vi "Test Drive OO.vi"() -> ()   [LabVIEW 2024]
uses:
  Ocean Optics Driver.lvclass
  Utilities/Fit/Peak Parameters.ctl
  Utilities/Fit/Multi-peak Parameters.ctl
  Ocean optics configuration.ctl
  LabActor/Recorders/Ruby Spectra/Ruby Spectra.lvclass
panel:
  in  "VISA resource name":refnum<visa-resource-name>="MayaPro"
  out "Spectral Waveform":T1(graph)
  in  "Ocean optics configuration":T2={"Integration time"=0.5, "Fit parameters"={"Function"=enum."Gauss", "Window width"=0.0, "Initial guess"={"Amplitude"=0.0, "Center"=690.0, "Width"=3.0}}, "Fit"=FALSE, "Auto-update params"=FALSE, "Save spectra"=FALSE, "Reference wavelengh"=694.123, "Background"=path ""} {"Reference wavelengh" format="%#_gnm"; "Fit parameters"."Initial guess"."Width" format="%#_gnm"; "Fit parameters"."Initial guess"."Center" format="%#_gnm"; "Fit parameters"."Window width" format="%#_6gnm"; "Integration time" format="%#_6ps"}
  in  "Device":string="MayaPro"
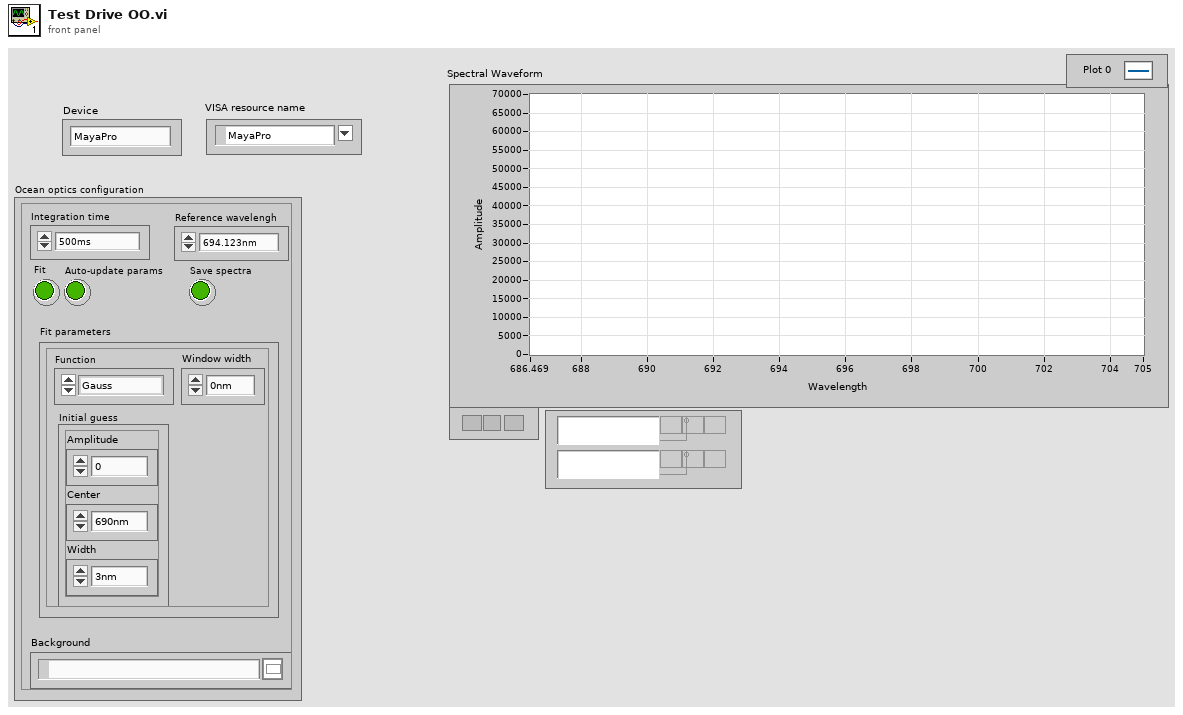
[diagram p1: front panel]
types:
  T1 = cluster{"Wavelength (nm)":dbl[], "Spectrum by Pixel Number":dbl[]}[]
  T2 = typedef "Ruby Spectra.lvclass/Ocean optics configuration.ctl" = cluster{"Integration time":dbl, "Fit parameters":T3, "Fit":bool, "Auto-update params":bool, "Save spectra":bool, "Reference wavelengh":dbl, "Background":path}
  T3 = typedef "Multi-peak Parameters.ctl" = cluster{"Function":enum16{"Gauss", "Lorentz"}, "Window width":dbl, "Initial guess":T4}
  T4 = typedef "Peak Parameters.ctl" = cluster{"Amplitude":dbl, "Center":dbl, "Width":dbl}
  T5 = cluster{"Wavelengths":dbl[], "Spectrum by Pixel Number":dbl[]}[]
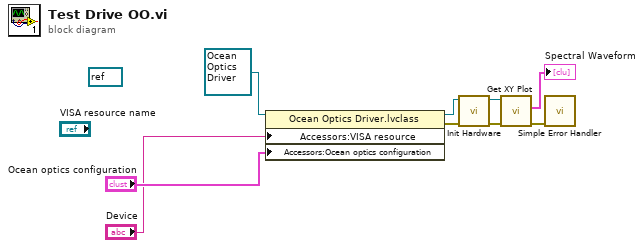
[diagram p0: block diagram]
diagram:
  (unwired) refnum<visa-resource-name> refnum ("VISA resource")
  n1 = property class="Ocean Optics Driver.lvclass"(reference=refnum<class "Ocean Optics Driver.lvclass"> refnum ("Ocean Optics Driver.lvclass"), "Accessors:VISA resource"="Device", "Accessors:Ocean optics configuration"="Ocean optics configuration") -> (reference out=w8:refnum<class "Ocean Optics Driver.lvclass">, error out=w7:errorcluster)  [unwired: 1 in]
  n2 = call-dynamic "Init Hardware.vi"("error in (no error)"=w7, "Ocean Optics Driver in"=w8) -> ("error out"=w4:errorcluster, "Ocean Optics Driver out"=w5:refnum<class "Ocean Optics Driver.lvclass">)  [unwired: 8 in]
  n3 = call-dynamic "Get XY Plot.vi"("error in (no error)"=w4, "Ocean Optics Driver in"=w5) -> ("error out"=w2:errorcluster, "Spectrum Graph"=→"Spectral Waveform":T5)  [unwired: 7 in, 1 out]
  n4 = call <vilib>:"Simple Error Handler.vi"("error in (no error)"=w2) -> ()  [unwired: 4 in, 5 out]
